vi "Throw JSON Error - Conversion Error.vi"(8 "error in (no error)":errorcluster, 9 "additional info":string, 10 "dest":string, 11 "source":string) -> (0 "error out":errorcluster)   [LabVIEW 2014, in "i3-json.lvlib"]
uses:
  i3-json.lvlib
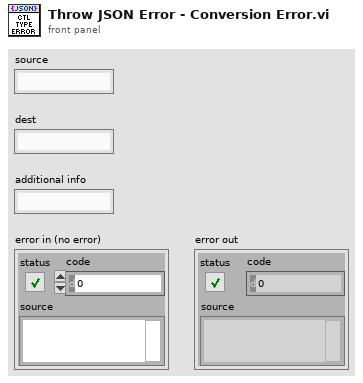
[diagram p1: front panel]
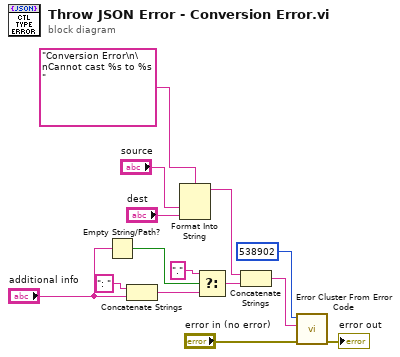
[diagram p0: block diagram]
diagram:
  n1 = Empty String/Path?(string/path="additional info") -> (empty?=w8:bool)
  n2 = Concatenate Strings(": " ("string"), "additional info") -> (w3:string)
  n3 = Format Into String(format string="Conversion Error\n\nCannot cast %s to %s " ("error message (\"\")"), "source", "dest") -> (resulting string=w2:string)  [unwired: 2 in, 1 out]
  n4 = Select(t="." ("datatype"), s=w8, f=w3) -> (s? t:f=w6:string)
  n5 = Concatenate Strings(w2, w6) -> (w1:string)
  n6 = call <vilib>:"Error Cluster From Error Code.vi"("error in (no error)"="error in (no error)", "error message (\"\")"=w1, "error code (0)"=538902) -> ("error out"=→"error out":errorcluster)  [unwired: 6 in]
